vi "KB-数据整合统计分析.vi"(10 "ALL Tolerance Param":string[][](table)=[["Null", "Null", "Null", "Null", "Null", "Null", "Null", "Null", "", ""], ["Null", "Null", "Null", "Null", "Null", "Null", "Null", "Null", "", ""], ["Null", "Null", "Null", "Null", "Null", "Null", "Null", "Null", "", ""], ["Null", "Null", "Null", "Null", "Null", "Null", "Null", "Null", "", ""], ["Null", "Null", "Null", "Null", "Null", "Null", "Null", "Null", "", ""], ["Null", "Null", "Null", "Null", "Null", "Null", "Null", "Null", "", ""], ["Null", "Null", "Null", "Null", "Null", "Null", "Null", "Null", "", ""], ["Null", "Null", "Null", "Null", "Null", "Null", "Null", "Null", "", ""], ["Null", "Null", "Null", "Null", "Null", "Null", "Null", "Null", "", ""], ["Null", "Null", "Null", "Null", "Null", "Null", "Null", "Null", "", ""], ["Null", "Null", "Null", "Null", "Null", "Null", "Null", "Null", "", ""], ["Null", "Null", "Null", "Null", "Null", "Null", "Null", "Null", "", ""], ["Null", "Null", "Null", "Null", "Null", "Null", "Null", "Null", "", ""], ["Null", "Null", "Null", "Null", "Null", "Null", "Null", "Null", "", ""], ["Null", "Null", "Null", "Null", "Null", "Null", "Null", "Null", "", ""], ["Null", "Null", "Null", "Null", "Null", "Null", "Null", "Null", "", ""], ["Null", "Null", "Null", "Null", "Null", "Null", "Null", "Null", "", ""], ["Null", "Null", "Null", "Null", "Null", "Null", "Null", "Null", "", ""], ["Null", "Null", "Null", "Null", "Null", "Null", "Null", "Null", "", ""], ["Null", "Null", "Null", "Null", "Null", "Null", "Null", "Null", "", ""], ["Null", "Null", "Null", "Null", "Null", "Null", "Null", "Null", "", ""], ["Null", "Null", "Null", "Null", "Null", "Null", "Null", "Null", "", ""], ["Null", "Null", "Null", "Null", "Null", "Null", "Null", "Null", "", ""], ["Null", "Null", "Null", "Null", "Null", "Null", "Null", "Null", "", ""], ["Null", "Null", "Null", "Null", "Null", "Null", "Null", "Null", "", ""], ["Null", "Null", "Null", "Null", "Null", "Null", "Null", "Null", "", ""], ["Null", "Null", "Null", "Null", "Null", "Null", "Null", "Null", "", ""], ["Null", "Null", "Null", "Null", "Null", "Null", "Null", "Null", "", ""], ["Null", "Null", "Null", "Null", "Null", "Null", "Null", "Null", "", ""], ["Null", "Null", "Null", "Null", "Null", "Null", "Null", "Null", "", ""], ["Null", "Null", "Null", "Null", "Null", "Null", "Null", "Null", "", ""]], 11 "Data Result":string[][](table)) -> (1 "Result":string, 2 "PASS/NG":bool, 3 "Data Result  Out":string[][](table))   [LabVIEW 2015]
panel:
  out "大小":i32
  out "数组 2":i32[](array[numeric])
  out "数组":string[](array[string])
  out "平面高度差上限":string[](array[string])
  out "平面高度差下限":string[](array[string])
  out "内环倾斜度差上限":string[](array[string])
  out "内环倾斜度差下限":string[](array[string])
  out "内外环高度差下限":string[](array[string])
  out "内外环高度差上限":string[](array[string])
  out "同心度下限":string[](array[string])
  out "同心度上限":string[](array[string])
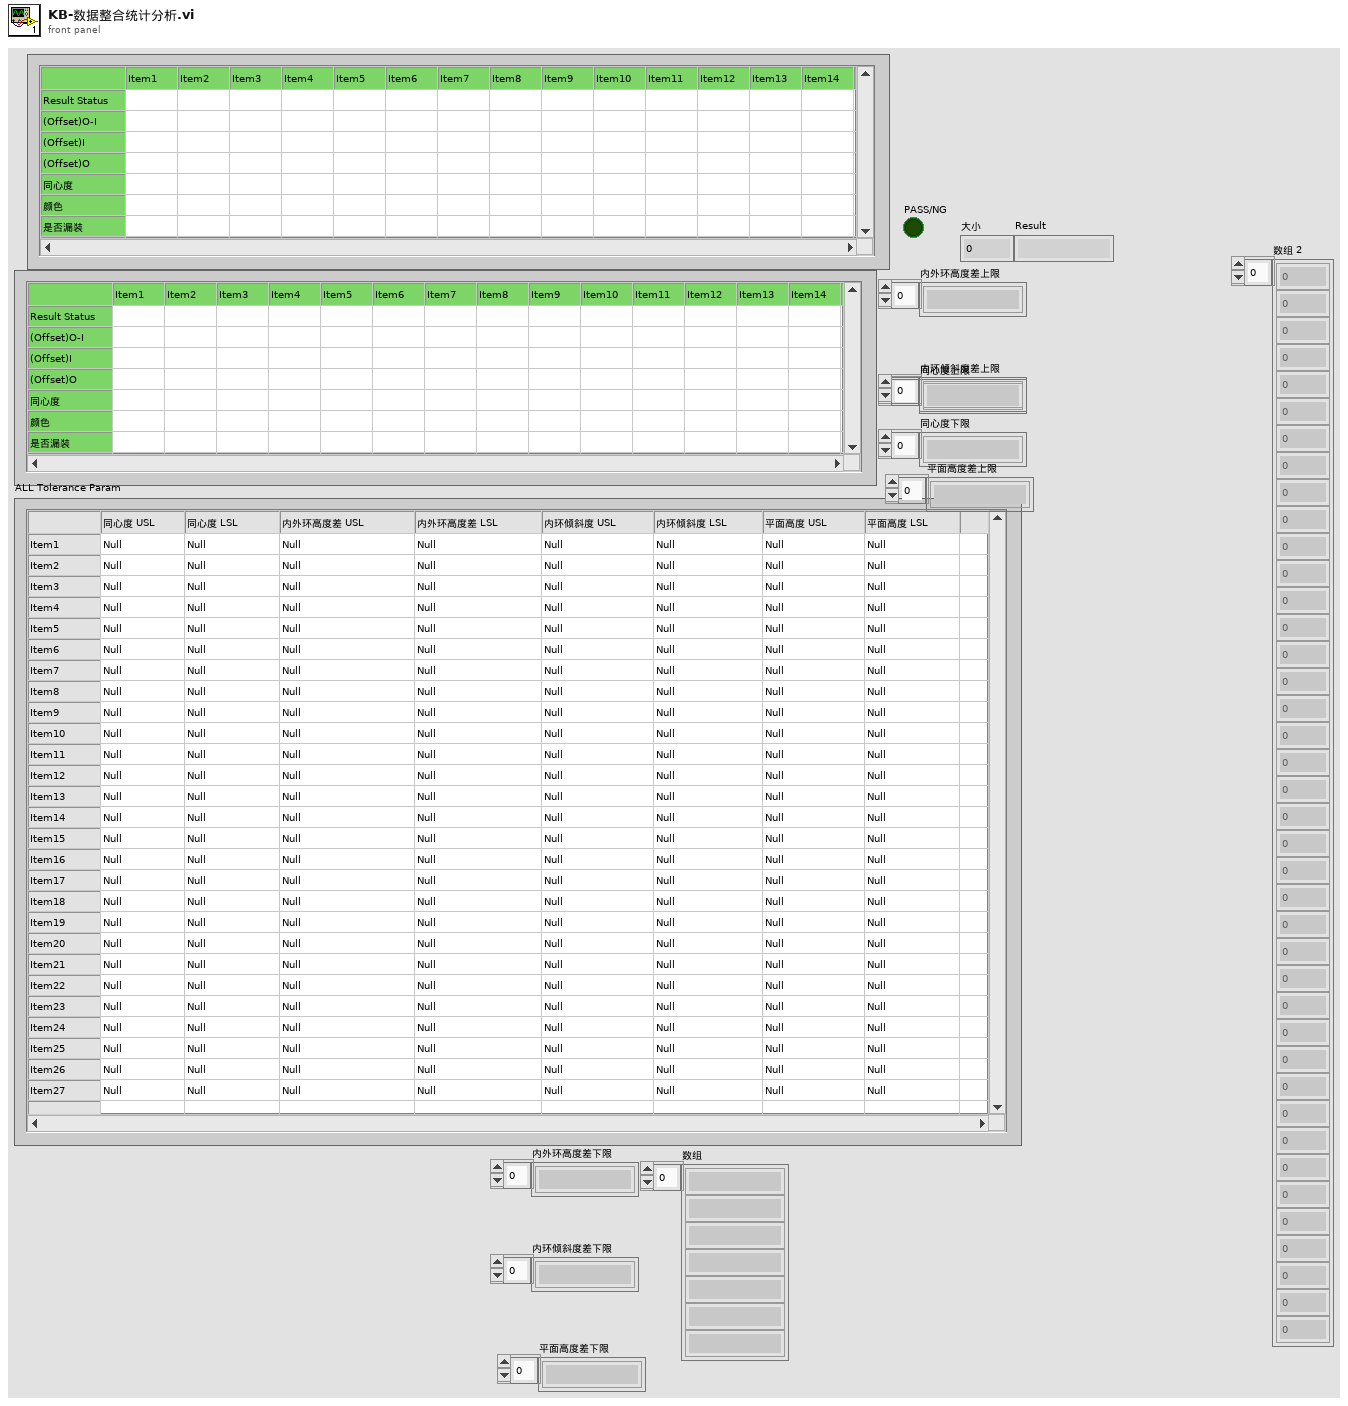
[diagram p1: front panel]
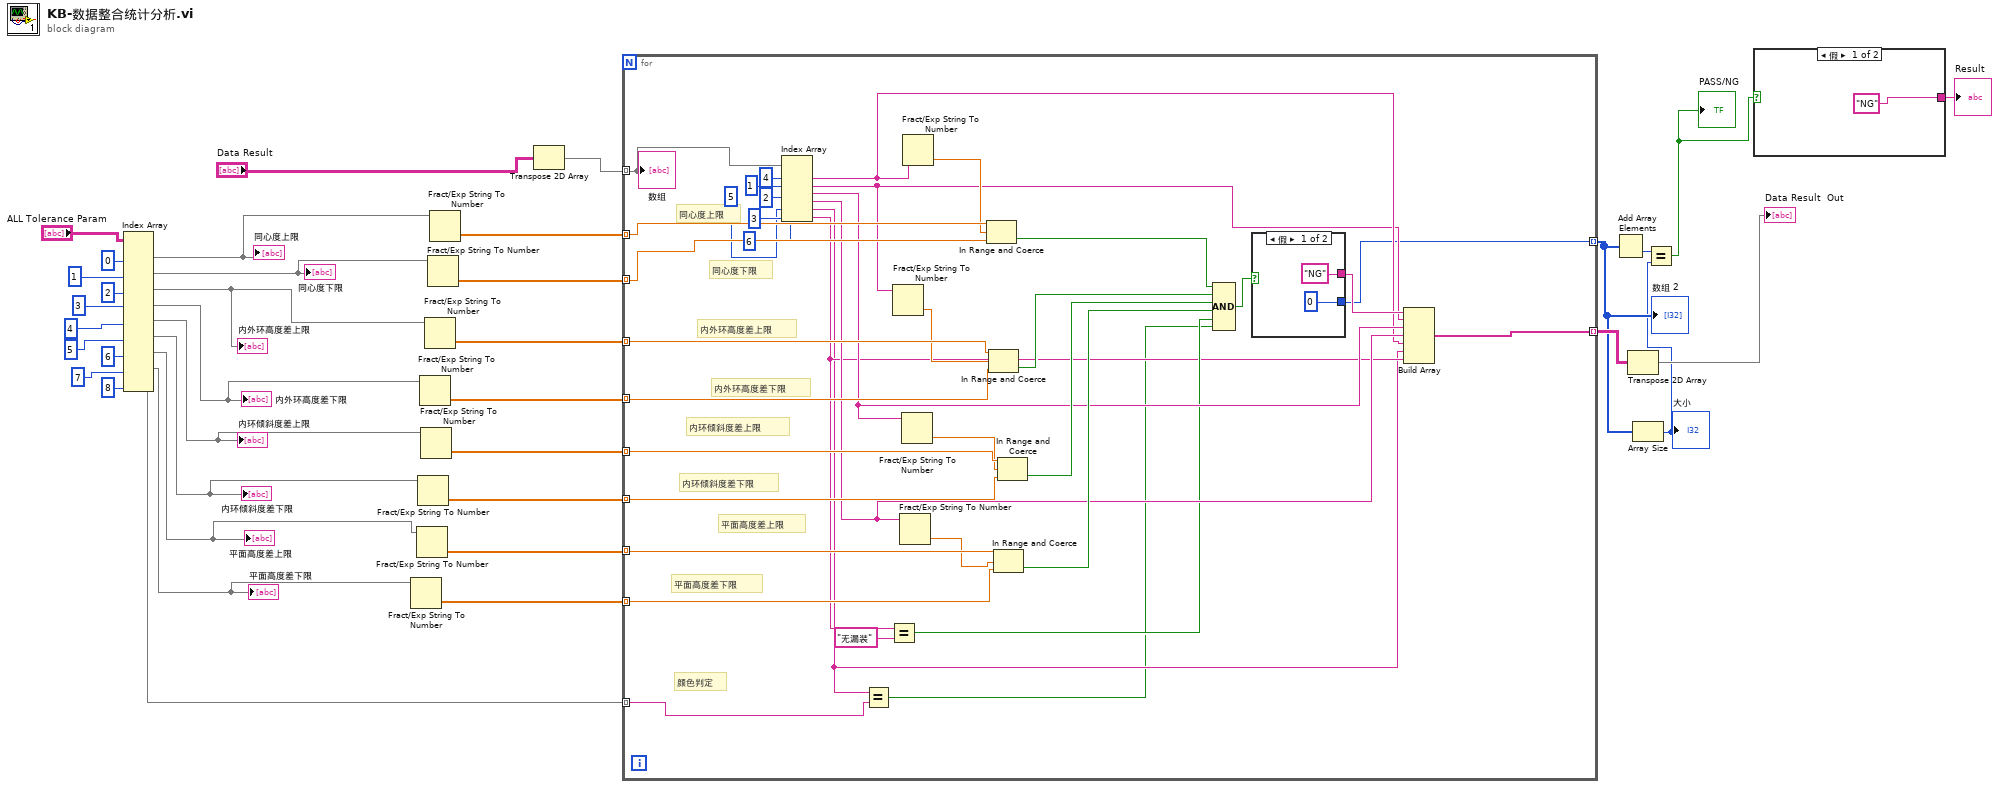
[diagram p0: block diagram]
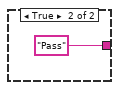
[diagram p2: hidden frame]
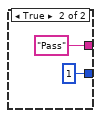
[diagram p3: hidden frame]
diagram:
  n1 = Index Array(array="ALL Tolerance Param", index (col) #1=0 ("禁用的索引 (列)"), index (col) #2=1 ("索引 (列)"), index (col) #3=2 ("索引 (列)"), index (col) #4=3 ("索引 (列)"), index (col) #5=4 ("索引 (列)"), index (col) #6=5 ("索引 (列)"), index (col) #7=6 ("索引 (列)"), index (col) #8=7 ("索引 (列)"), index (col) #9=8 ("索引 (列)")) -> (element #1=w25:string[], element #2=w24:string[], element #3=w23:string[], element #4=w22:string[], element #5=w21:string[], element #6=w20:string[], element #7=w19:string[], element #8=w18:string[], element #9=w6:string[])  [unwired: 9 in]
  "同心度上限" <- w25
  "同心度下限" <- w24
  "内外环高度差上限" <- w23
  "内外环高度差下限" <- w22
  "内环倾斜度差上限" <- w21
  "内环倾斜度差下限" <- w20
  "平面高度差上限" <- w19
  "平面高度差下限" <- w18
  n2 = Fract/Exp String To Number(string=w18) -> (number=w10:dbl[])  [unwired: 3 in, 1 out]
  n3 = Fract/Exp String To Number(string=w19) -> (number=w11:dbl[])  [unwired: 3 in, 1 out]
  n4 = Fract/Exp String To Number(string=w20) -> (number=w12:dbl[])  [unwired: 3 in, 1 out]
  n5 = Fract/Exp String To Number(string=w22) -> (number=w14:dbl[])  [unwired: 3 in, 1 out]
  n6 = Fract/Exp String To Number(string=w21) -> (number=w13:dbl[])  [unwired: 3 in, 1 out]
  n7 = Fract/Exp String To Number(string=w23) -> (number=w15:dbl[])  [unwired: 3 in, 1 out]
  n8 = Fract/Exp String To Number(string=w24) -> (number=w16:dbl[])  [unwired: 3 in, 1 out]
  n9 = Fract/Exp String To Number(string=w25) -> (number=w17:dbl[])  [unwired: 3 in, 1 out]
  n10 = Transpose 2D Array(2D array="Data Result") -> (transposed array=w26:string[][])
  n11 = for {
    tunnel: w26 -> [w65] mode=indexing
    tunnel: w17 -> [w73] mode=indexing
    tunnel: w16 -> [w72] mode=indexing
    tunnel: w15 -> [w71] mode=indexing
    tunnel: w14 -> [w70] mode=indexing
    tunnel: w13 -> [w69] mode=indexing
    tunnel: w12 -> [w68] mode=indexing
    tunnel: w11 -> [w67] mode=indexing
    tunnel: w10 -> [w66] mode=indexing
    tunnel: [w43] -> w9 mode=indexing
    tunnel: w6 -> [w39] mode=indexing
    tunnel: [w40] -> w5 mode=indexing
    # "颜色判定"
    # "平面高度差下限"
    # "平面高度差上限"
    # "内环倾斜度差下限"
    # "内环倾斜度差上限"
    # "内外环高度差下限"
    # "内外环高度差上限"
    # "同心度下限"
    # "同心度上限"
    n12 = Index Array(array=w65, index #1=4 ("索引"), index #2=1 ("索引"), index #3=2 ("索引"), index #4=3 ("索引"), index #5=5 ("索引"), index #6=6 ("索引")) -> (element #1=w42:string, element #2=w41:string, element #3=w52:string, element #4=w49:string, element #5=w38:string, element #6=w44:string)
    n13 = Equal?(x=w38, y=w39) -> (x = y?=w37:bool)
    n14 = Equal?(x=w44, y="无漏装") -> (x = y?=w45:bool)
    n15 = Fract/Exp String To Number(string=w41) -> (number=w55:dbl)  [unwired: 3 in, 1 out]
    n16 = Fract/Exp String To Number(string=w49) -> (number=w50:dbl)  [unwired: 3 in, 1 out]
    n17 = Fract/Exp String To Number(string=w52) -> (number=w53:dbl)  [unwired: 3 in, 1 out]
    n18 = Fract/Exp String To Number(string=w42) -> (number=w63:dbl)  [unwired: 3 in, 1 out]
    n19 = In Range and Coerce(upper limit=w73, x=w63, lower limit=w72) -> (In Range?=w62:bool)  [unwired: 1 out]
    n20 = In Range and Coerce(upper limit=w71, x=w55, lower limit=w70) -> (In Range?=w61:bool)  [unwired: 1 out]
    n21 = In Range and Coerce(upper limit=w67, x=w50, lower limit=w66) -> (In Range?=w59:bool)  [unwired: 1 out]
    n22 = In Range and Coerce(upper limit=w69, x=w53, lower limit=w68) -> (In Range?=w60:bool)  [unwired: 1 out]
    n23 = Compound Arithmetic op=AND ("复合运算")(w62, w61, w60, w59, w45, w37) -> (w58:bool)
    n24 = case shown="假" w58 {
      tunnel: ["NG" "Pass"] -> w56
      tunnel: [0 1] -> w40
      frame False {
      }
      frame True {
      }
    }
    n25 = Build Array(w56, w41, w52, w49, w42, w38, w44) -> (w43:string[])
    "数组" <- w65
  }
  "数组 2" <- w5
  n26 = Add Array Elements(numeric array=w5) -> (sum=w4:i32)
  n27 = Transpose 2D Array(2D array=w9) -> (transposed array=→"Data Result  Out":string[][])
  n28 = Array Size(array=w5) -> (size(s)=w3:i32)
  "大小" <- w3
  n29 = Equal?(x=w4, y=w3) -> (x = y?=w2:bool)
  "PASS/NG" <- w2
  n30 = case shown="假" w2 {
    tunnel: ["NG" "Pass"] -> w1
    frame False {
    }
    frame True {
    }
  }
  "Result" <- w1
